vi "StringList.Reset.vi"(8 "error in (no error)":errorcluster, 11 "StringList in":refnum<class "StringList.lvclass">) -> (0 "error out":errorcluster, 2 "Items Out":string[](array[string]), 3 "StringList out":refnum<class "StringList.lvclass">)   [LabVIEW 2024, in "StringList.lvclass"]
uses:
  StringList.lvclass
  StringList.lvclass/StringList.ctl
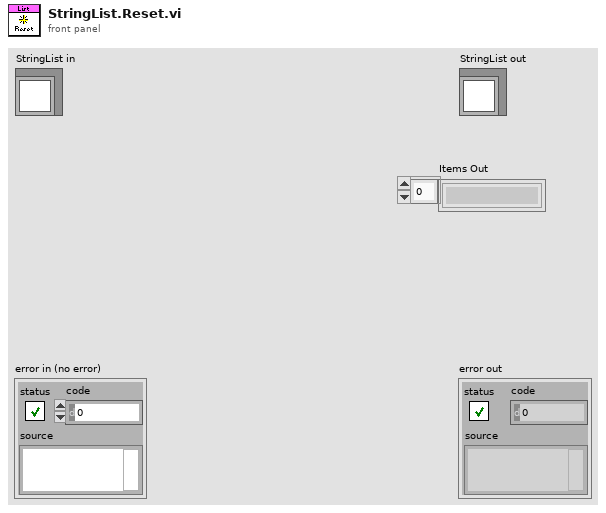
[diagram p1: front panel]
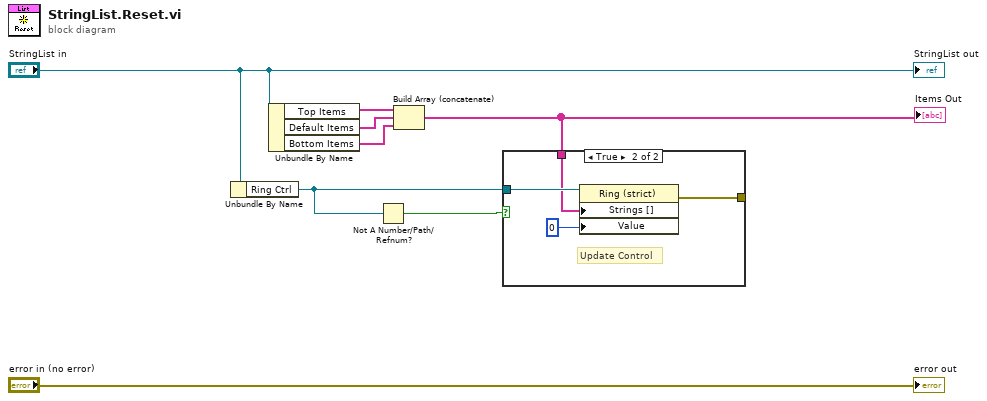
[diagram p0: block diagram]
diagram:
  n1 = Unbundle By Name("StringList in") -> ("Ring Ctrl"=w6:refnum<vi>)
  n2 = Unbundle By Name("StringList in") -> ("Top Items"=w5:string[], "Default Items"=w4:string[], "Bottom Items"=w3:string[])
  n3 = Not A Number/Path/Refnum?(number/path/refnum=w6) -> (NaN/Path/Refnum?=w2:bool)
  n4 = Build Array (concatenate)(w5, w4, w3) -> (w7:string[])
  "Items Out" <- w7
  n5 = case shown="True" w2 {
    tunnel: w6 -> [_ w12]
    tunnel: w7 -> [_ w10]
    tunnel: [_ w9] -> _
    frame False {
    }
    frame True {
      # "Update Control"
      n6 = property class="Ring (strict)"(reference=w12, "Strings []"=w10, "Value"=u16 0) -> (error out=w9:errorcluster)  [unwired: 1 in, 1 out]
    }
  }
  "error out" <- "error in (no error)"
  "StringList out" <- "StringList in"
